vi "Vacuum Test - Step 3.vi"(7 "Step":i32, 8 "error in":errorcluster, 9 "Test Results In":T9, 10 "PAS In":T8 caption="Gas", 11 "Test Configuration":T1) -> (0 "error out":errorcluster, 1 "Test Results Out":T9, 2 "PAS Out":T8 caption="Gas", 3 "Test Configuration Out":T1)   [LabVIEW 2015]
uses:
  CAN Communication/PAS/Typedefs/Session Handle.ctl
  CAN Communication/PAS/PAS.lvclass
  Controls/Test Results.ctl
  Controls/Step Result.ctl
  Controls/Test Configuration.ctl
  Controls/Vacuum Test.ctl
  Controls/Test Timing.ctl
  Controls/Vaccum Thresholds.ctl
  Controls/Helium Test.ctl
  Controls/Helium Thresholds.ctl
  Controls/Functional Test.ctl
  CAN Communication/PAS/Typedefs/Valves.ctl
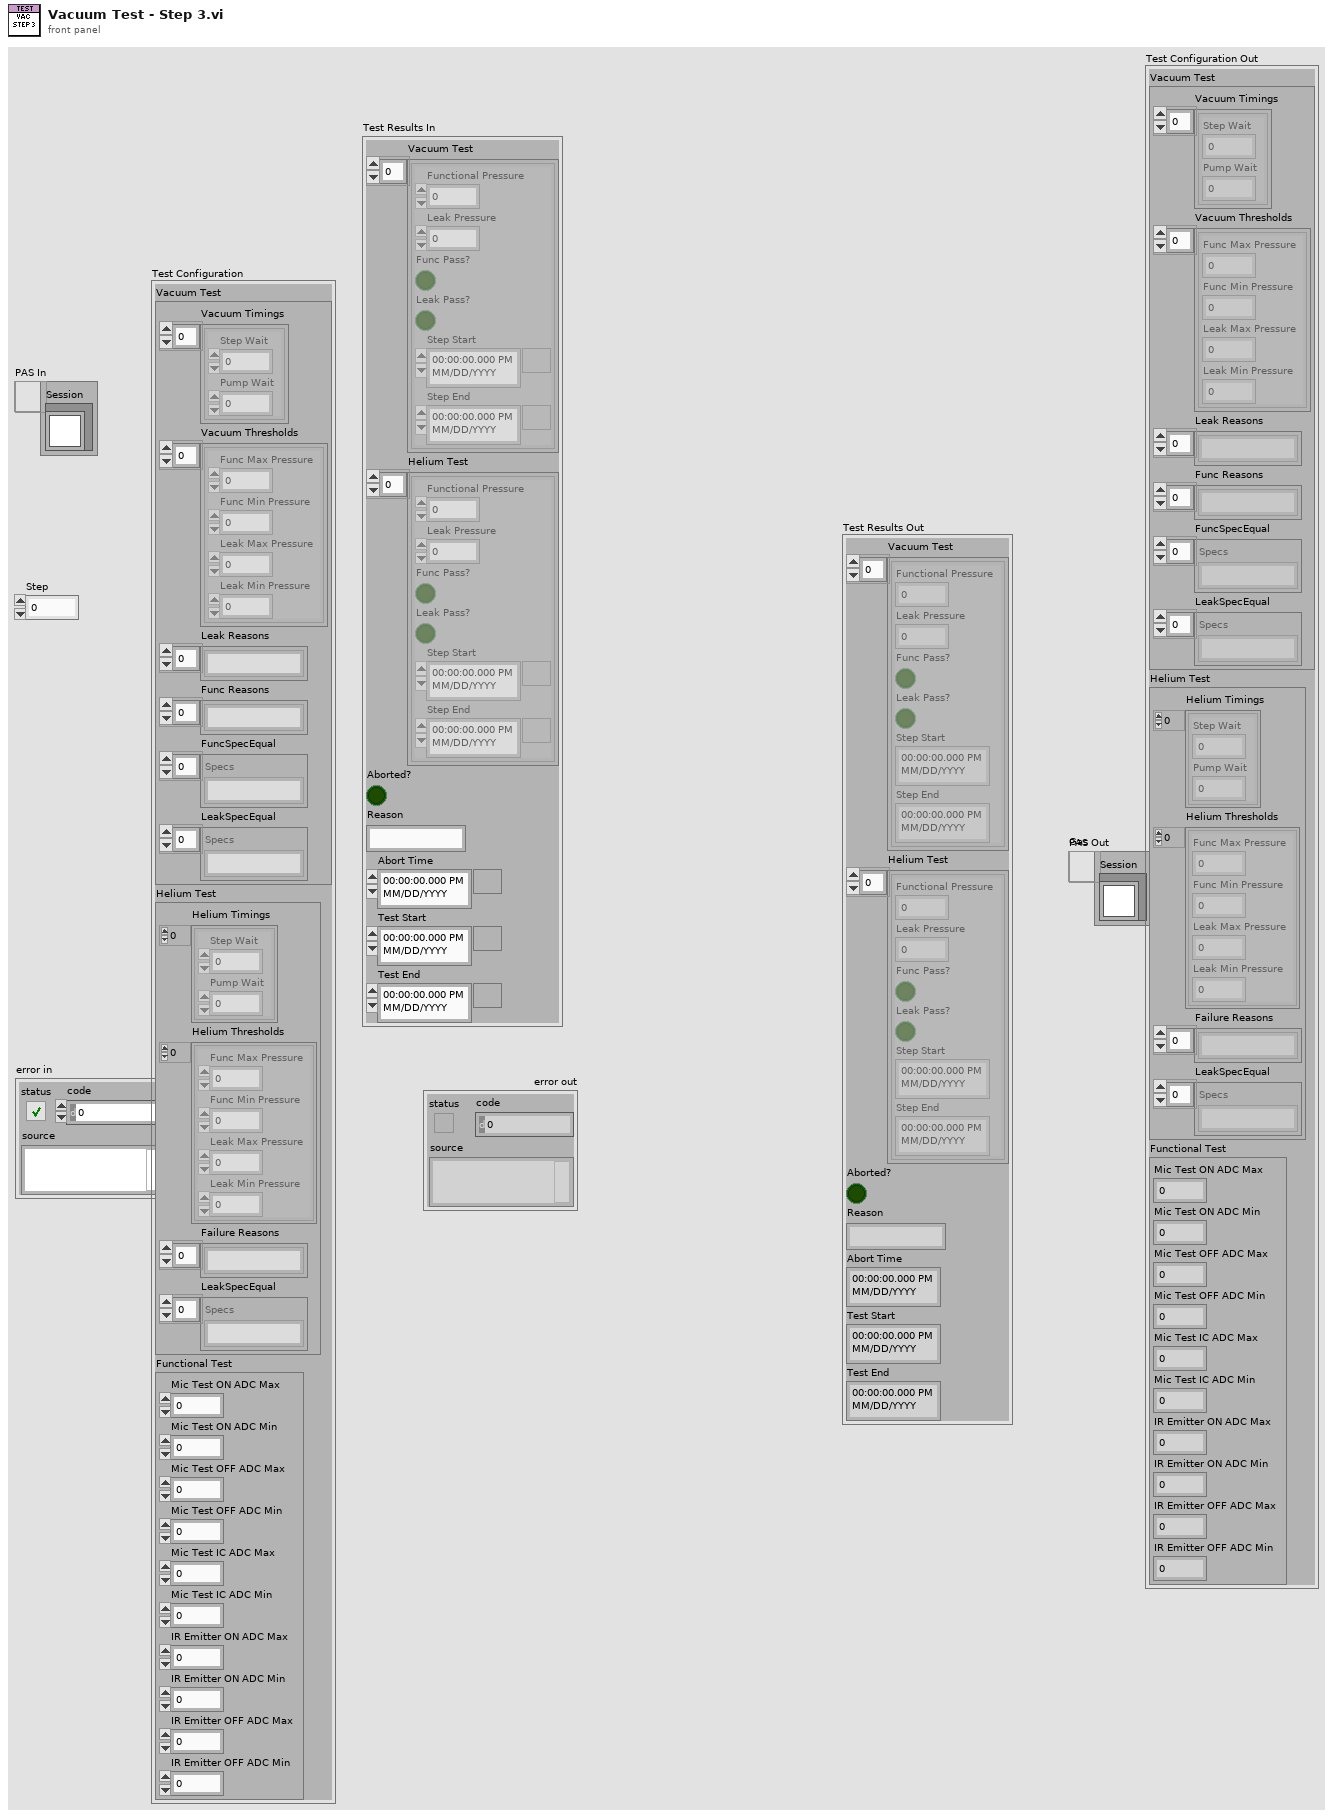
[diagram p1: front panel]
types:
  T1 = typedef "Test Configuration.ctl" = cluster{"Vacuum Test":T2, "Helium Test":T5, "Functional Test":T7}
  T2 = typedef "Vacuum Test.ctl" = cluster{"Vacuum Timings":T3[], "Vacuum Thresholds":T4[], "Leak Reasons":string[], "Func Reasons":string[], "FuncSpecEqual":string[], "LeakSpecEqual":string[]}
  T3 = typedef "Test Timing.ctl" = cluster{"Step Wait":dbl, "Pump Wait":dbl}
  T4 = typedef "Vaccum Thresholds.ctl" = cluster{"Func Max Pressure":dbl, "Func Min Pressure":dbl, "Leak Max Pressure":dbl, "Leak Min Pressure":dbl}
  T5 = typedef "Helium Test.ctl" = cluster{"Helium Timings":T3[], "Helium Thresholds":T6[], "Failure Reasons":string[], "LeakSpecEqual":string[]}
  T6 = typedef "Helium Thresholds.ctl" = cluster{"Func Max Pressure":dbl, "Func Min Pressure":dbl, "Leak Max Pressure":dbl, "Leak Min Pressure":dbl}
  T7 = typedef "Functional Test.ctl" = cluster{"Mic Test ON ADC Max":dbl, "Mic Test ON ADC Min":dbl, "Mic Test OFF ADC Max":dbl, "Mic Test OFF ADC Min":dbl, "Mic Test IC ADC Max":dbl, "Mic Test IC ADC Min":dbl, "IR Emitter ON ADC Max":dbl, "IR Emitter ON ADC Min":dbl, "IR Emitter OFF ADC Max":dbl, "IR Emitter OFF ADC Min":dbl}
  T8 = typedef "PAS.lvclass/Session Handle.ctl" = refnum<data-value>
  T9 = typedef "Test Results.ctl" = cluster{"Vacuum Test":T10[], "Helium Test":T10[], "Aborted?":bool, "Reason":string, "Abort Time":timestamp, "Test Start":timestamp, "Test End":timestamp}
  T10 = typedef "Step Result.ctl" = cluster{"Functional Pressure":dbl, "Leak Pressure":dbl, "Func Pass?":bool, "Leak Pass?":bool, "Step Start":timestamp, "Step End":timestamp}
  T11 = typedef "PAS.lvclass/Valves.ctl" = u16
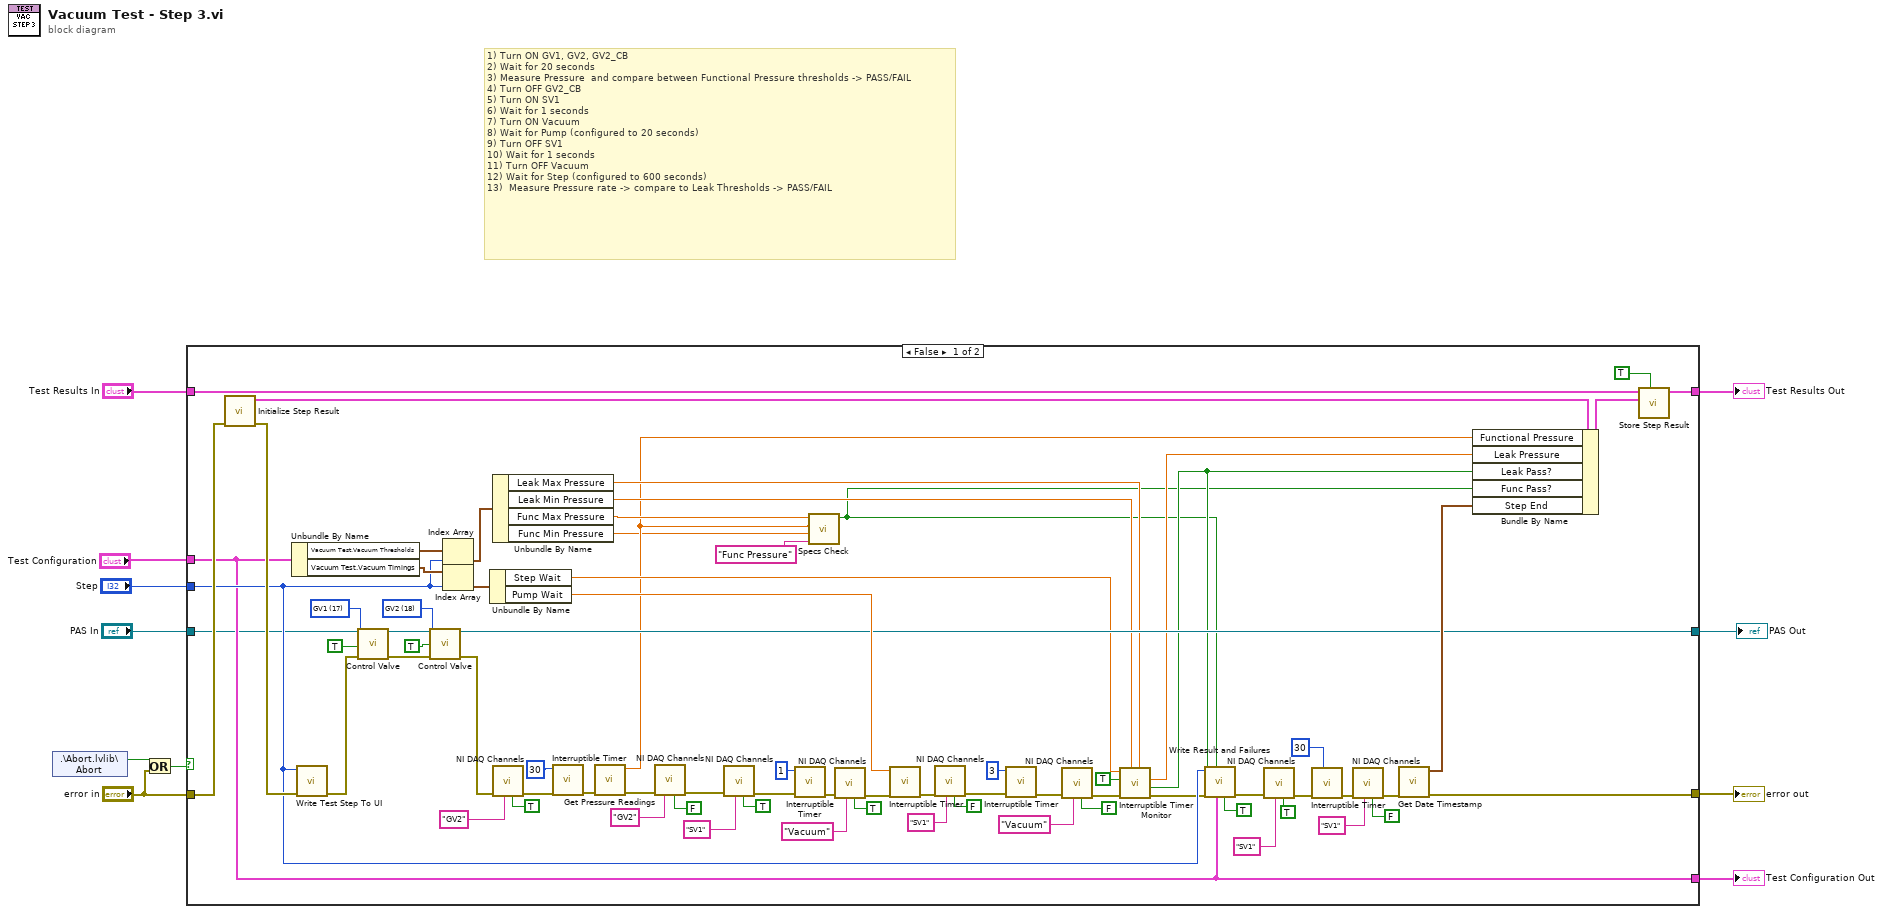
[diagram p0: block diagram]
diagram:
  # "1) Turn ON GV1, GV2, GV2_CB\n2) Wait for 20 seconds\n3) Measure Pressure  and compare between Functional Pressure thresholds -> PASS/FAIL\n4) Turn OFF GV2_CB\n5) Turn ON SV1\n6) Wait for 1 seconds\n7) Turn ON Vacuum\n8) Wait for Pump (configured to 20 seconds)\n9) Turn OFF SV1\n10) Wait for 1 seconds\n11) Turn OFF Vacuum\n12) Wait for Step (configured to 600 seconds)\n13)  Measure Pressure rate -> compare to Leak Thresholds -> PASS/FAIL"
  n1 = shared-variable ".\\Abort.lvlib\\Abort"() -> (w10:bool)  [unwired: 1 in, 1 out]
  n2 = Or(x=w10, y="error in") -> (x .or. y?=w9:bool)
  n3 = case shown="False" w9 {
    tunnel: "error in" -> [w85 w88]
    tunnel: "Test Results In" -> [w82 w89]
    tunnel: [w83 w89] -> w7
    tunnel: [w26 w88] -> w6
    tunnel: "Test Configuration" -> [w64 w87]
    tunnel: "Step" -> [w72 _]
    tunnel: [w64 w87] -> w1
    tunnel: [w42 w86] -> w3
    tunnel: "PAS In" -> [w62 w86]
    frame False {
      w54 = T11 18 items=["GV1"=17, "GV2"=18, "GV3"=19, "GV4"=20] ("Valves")
      w55 = T11 17 items=["GV1"=17, "GV2"=18, "GV3"=19, "GV4"=20] ("Valves")
      n4 = call "Initialize Step Result.vi"("error in (no error)"=w85) -> ("error out"=w84:errorcluster, "New Step Result"=w81:T10)  [unwired: 8 in, 1 out]
      n5 = Unbundle By Name(w64) -> ("Vacuum Test.Vacuum Thresholds"=w78:T4[], "Vacuum Test.Vacuum Timings"=w77:T3[])
      n6 = call "Write Test Step To UI.vi"("error in (no error)"=w84, "Step"=w72) -> ("error out"=w57:errorcluster)  [unwired: 9 in]
      n7 = call "Control Valve.vi"("Session Handle in"=w62, "Valves"=w55, "Energize?"=TRUE, "error in (no error)"=w57) -> ("Session Handle out"=w60:T8, "error out"=w58:errorcluster)  [unwired: 8 in, 2 out]
      n8 = call "Control Valve.vi"("Session Handle in"=w60, "Valves"=w54, "Energize?"=TRUE, "error in (no error)"=w58) -> ("Session Handle out"=w42:T8, "error out"=w56:errorcluster)  [unwired: 8 in, 2 out]
      n9 = Index Array(array=w78, index=w72) -> (element=w74:T4)
      n10 = Index Array(array=w77, index=w72) -> (element=w76:T3)
      n11 = Unbundle By Name(w76) -> ("Step Wait"=w40:dbl, "Pump Wait"=w49:dbl)
      n12 = Unbundle By Name(w74) -> ("Leak Max Pressure"=w38:dbl, "Leak Min Pressure"=w39:dbl, "Func Max Pressure"=w15:dbl, "Func Min Pressure"=w13:dbl)
      n13 = call "NI DAQ Channels.vi"("Control"=TRUE ("State"), "Channel"="GV2", "error in (no error)"=w56) -> ("error out"=w70:errorcluster)  [unwired: 7 in, 1 out]
      n14 = call "Interruptible Timer.vi"("error in (no error)"=w70, "Wait (s)"=30) -> ("error out"=w63:errorcluster)  [unwired: 7 in, 2 out]
      n15 = call "Get Pressure Readings.vi"("error in (no error)"=w63) -> ("error out"=w53:errorcluster, "NI-DAQ Pressure"=w14:dbl)  [unwired: 7 in, 2 out]
      n16 = call "NI DAQ Channels.vi"("Control"=FALSE ("State"), "Channel"="GV2", "error in (no error)"=w53) -> ("error out"=w51:errorcluster)  [unwired: 7 in, 1 out]
      n17 = call "NI DAQ Channels.vi"("Control"=TRUE ("State"), "Channel"="SV1", "error in (no error)"=w51) -> ("error out"=w67:errorcluster)  [unwired: 7 in, 1 out]
      n18 = call "Interruptible Timer.vi"("error in (no error)"=w67, "Wait (s)"=1) -> ("error out"=w65:errorcluster)  [unwired: 7 in, 2 out]
      n19 = call "Specs Check.vi"("parameter"="Func Pressure", "lower limit"=w13, "x"=w14, "upper limit"=w15) -> ("In Range?"=w16:bool)  [unwired: 6 in, 1 out]
      n20 = call "NI DAQ Channels.vi"("Control"=TRUE ("State"), "Channel"="Vacuum", "error in (no error)"=w65) -> ("error out"=w50:errorcluster)  [unwired: 7 in, 1 out]
      n21 = call "Interruptible Timer.vi"("error in (no error)"=w50, "Wait (s)"=w49) -> ("error out"=w44:errorcluster)  [unwired: 7 in, 2 out]
      n22 = call "NI DAQ Channels.vi"("Control"=FALSE ("State"), "Channel"="SV1", "error in (no error)"=w44) -> ("error out"=w47:errorcluster)  [unwired: 7 in, 1 out]
      n23 = call "Interruptible Timer.vi"("error in (no error)"=w47, "Wait (s)"=3) -> ("error out"=w48:errorcluster)  [unwired: 7 in, 2 out]
      n24 = call "NI DAQ Channels.vi"("Control"=FALSE ("State"), "Channel"="Vacuum", "error in (no error)"=w48) -> ("error out"=w41:errorcluster)  [unwired: 7 in, 1 out]
      n25 = call "Interruptible Timer Monitor.vi"("Max"=w38, "Min"=w39, "error in (no error)"=w41, "Update UI?"=TRUE, "Wait (s)"=w40) -> ("error out"=w28:errorcluster, "In Range?"=w36:bool, "Leak Rate"=w37:dbl)  [unwired: 2 in, 2 out]
      n26 = call "Write Result and Failures.vi"("Vacuum?"=TRUE, "Leak"=w36, "Test Configuration"=w64, "Func"=w16, "error in (no error)"=w28, "Step"=w72) -> ("error out"=w27:errorcluster)  [unwired: 5 in]
      n27 = call "NI DAQ Channels.vi"("Control"=TRUE ("State"), "Channel"="SV1", "error in (no error)"=w27) -> ("error out"=w34:errorcluster)  [unwired: 7 in, 1 out]
      n28 = call "Interruptible Timer.vi"("error in (no error)"=w34, "Wait (s)"=30) -> ("error out"=w32:errorcluster)  [unwired: 7 in, 2 out]
      n29 = call "NI DAQ Channels.vi"("Control"=FALSE ("State"), "Channel"="SV1", "error in (no error)"=w32) -> ("error out"=w30:errorcluster)  [unwired: 7 in, 1 out]
      n30 = call "Get Date Timestamp.vi"("error in (no error)"=w30) -> ("error out"=w26:errorcluster, "current time"=w79:timestamp)  [unwired: 9 in]
      n31 = Bundle By Name(cluster=w81, "Functional Pressure"=w14, "Leak Pressure"=w37, "Leak Pass?"=w36, "Func Pass?"=w16, "Step End"=w79) -> (w80:T10)
      n32 = call "Store Step Result.vi"("Vacuum?"=TRUE, "Step Result"=w80, "Test Results In"=w82) -> ("Test Results Out"=w83:T9)  [unwired: 8 in]
    }
    frame True {
    }
  }
  "error out" <- w6
  "Test Results Out" <- w7
  "PAS Out" <- w3
  "Test Configuration Out" <- w1
